vi "BuildMenu3.vi"(8 "Click Type":T6, 9 "Point":T7, 10 "XRef":refnum<vi>, 11 "State In":T10) -> (1 "Show Standard Items? (Popup click only)":bool=TRUE, 2 "Menu Specification":T9)   [LabVIEW 2012, in "CThread.lvlib" / "CThread VI Terminal Node.xnode"]
doc: "This ability VI is used to describe the menu LabVIEW will display in response to a popup (right) click or a ShowMenu reply from OperateClick.\n \n Click Type is the type of click that led to this call of the ability. Point is the location of the user's popup click, and is relative to the top-left corner of your XNode's bounds. You may use this point to make your popup sensitive to the location that was clicked. Show Standard Items? is applicable only if Click Type is Popup, and tells LabVIEW whether it should include the standard popup items that are included on every node in LabVIEW.\n \n Menu Specification is an array of clusters describing the menu.\n Item: A string that will appear in the menu.\n Id: A string that identifies this item and will be passed to SelectMenu3.\n StartSub: The current string will be the header for a pull right menu.\n EndSub: The current string will be the last item in a pull right menu.\n Checked: The current item will have a check mark next to it.\n Disabled: The current item will be diabled and greyed out.\n Separator: The current item will be a separator. Item string is not displayed.\n Help: The text that should be displayed in context help when this menu item is hovered over. This functionality is currently not implemented.\n \n The index from this array will be an input to SelectMenu3.\n \n Remember to localize the strings in your menu.\n\nDefault behavior: Only show standard items for a popup click, show nothing for operate click.\n\nThis ability does not provide UI and OS messages are not handled.\n\nSee also: SelectMenu3"
uses:
  CThread VI Terminal Node.xnode
  State.ctl
  <vilib>/XNodeSupport/XNodeMenuSpecs3.ctl
  <vilib>/XNodeSupport/XNodeMenuSpec3.ctl
  <vilib>/XNodeSupport/XNodeString.ctl
  <vilib>/XNodeSupport/XNodeBool.ctl
  <vilib>/XNodeSupport/XNodeStandardHelpInfo.ctl
  <vilib>/XNodeSupport/XNodePath.ctl
  <vilib>/XNodeSupport/XNodePoint.ctl
  <vilib>/XNodeSupport/XNodeInt.ctl
  <vilib>/XNodeSupport/XNodeClickTypes.ctl
  <vilib>/XNodeSupport/XNodeRect32.ctl
  <vilib>/XNodeSupport/NI_XNodeSupport.lvlib
panel:
  in  "Menu Item 3":T1
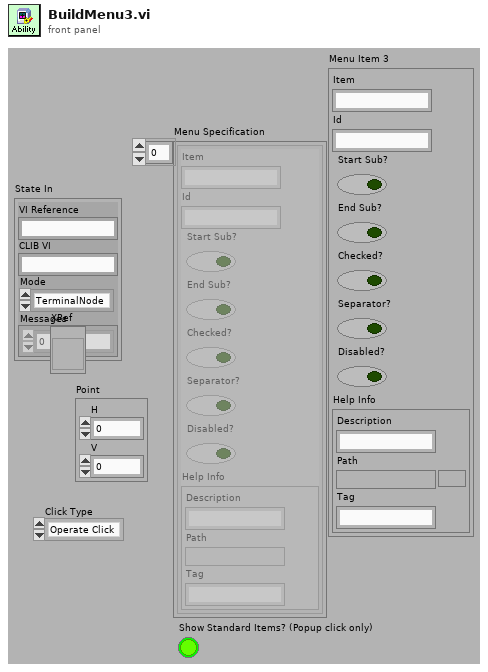
[diagram p1: front panel]
types:
  T1 = typedef "NI_XNodeSupport.lvlib/XNodeMenuSpec3.ctl" = cluster{"Item":T2, "Id":T2, "Start Sub?":T3, "End Sub?":T3, "Checked?":T3, "Separator?":T3, "Disabled?":T3, "Help Info":T4}
  T2 = typedef "NI_XNodeSupport.lvlib/XNodeString.ctl" = string
  T3 = typedef "NI_XNodeSupport.lvlib/XNodeBool.ctl" = bool
  T4 = typedef "NI_XNodeSupport.lvlib/XNodeStandardHelpInfo.ctl" = cluster{"Description":T2, "Path":T5, "Tag":T2}
  T5 = typedef "NI_XNodeSupport.lvlib/XNodePath.ctl" = path
  T6 = typedef "NI_XNodeSupport.lvlib/XNodeClickTypes.ctl" = enum32{"Operate Click", "Popup Click"}
  T7 = typedef "NI_XNodeSupport.lvlib/XNodePoint.ctl" = cluster{"H":T8, "V":T8}
  T8 = typedef "NI_XNodeSupport.lvlib/XNodeInt.ctl" = i32
  T9 = typedef "NI_XNodeSupport.lvlib/XNodeMenuSpecs3.ctl" = T1[]
  T10 = typedef "CThread.lvlib/CThread VI Terminal Node.xnode/State.ctl" = cluster{"VI Reference":string, "CLIB VI":string, "Mode":enum16{"TerminalNode", "AdaptorNode"}, "Messages":u8[]}
  T11 = typedef "NI_XNodeSupport.lvlib/XNodeRect32.ctl" = cluster{"Left":T8, "Top":T8, "Right":T8, "Bottom":T8}
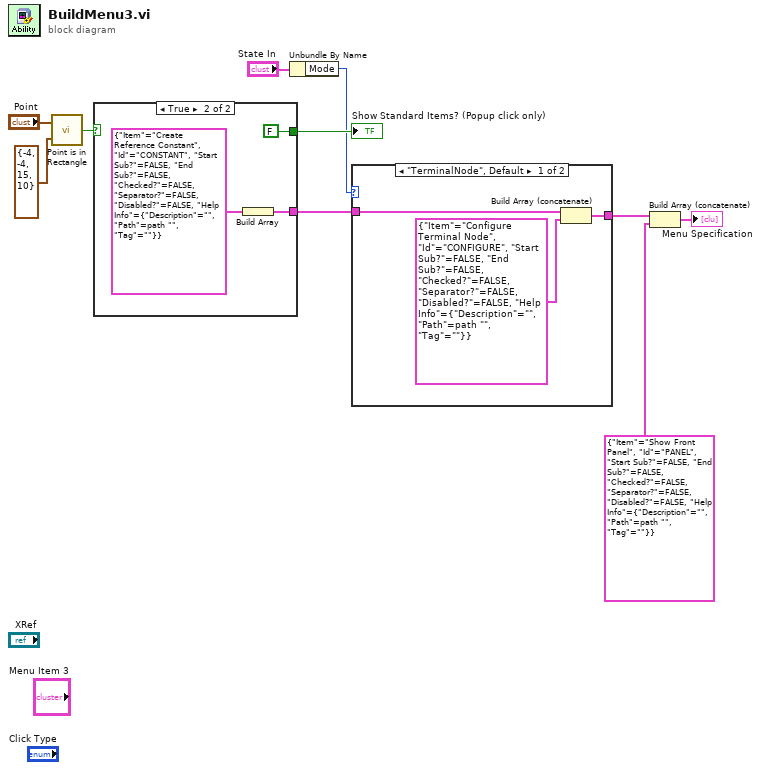
[diagram p0: block diagram]
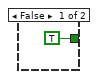
[diagram p3: hidden frame]
diagram:
  n1 = call "Point is in Rectangle.vi"("Bounds"=T11 {"Left"=-4, "Top"=-4, "Right"=15, "Bottom"=10}, "Point"="Point") -> ("In Bounds?"=w9:bool)
  n2 = case shown="True" w9 {
    tunnel: [TRUE FALSE] -> w7
    tunnel: [_ w12] -> w4
    frame False {
    }
    frame True {
      n3 = Build Array(T1 {"Item"="Create Reference Constant", "Id"="CONSTANT", "Start Sub?"=FALSE, "End Sub?"=FALSE, "Checked?"=FALSE, "Separator?"=FALSE, "Disabled?"=FALSE, "Help Info"={"Description"="", "Path"=path "", "Tag"=""}} ("Menu Item 3")) -> (w12:T1[])
    }
  }
  "Show Standard Items? (Popup click only)" <- w7
  n4 = Unbundle By Name("State In") -> ("Mode"=w5:enum16{"TerminalNode", "AdaptorNode"})
  n5 = case shown="\"TerminalNode\", Default" w5 {
    tunnel: w4 -> [w17 w18]
    tunnel: [w15 w18] -> w3
    frame "TerminalNode", Default {
      n6 = Build Array (concatenate)(w17, T1 {"Item"="Configure Terminal Node", "Id"="CONFIGURE", "Start Sub?"=FALSE, "End Sub?"=FALSE, "Checked?"=FALSE, "Separator?"=FALSE, "Disabled?"=FALSE, "Help Info"={"Description"="", "Path"=path "", "Tag"=""}} ("Menu Item 3")) -> (w15:T1[])
    }
    frame "AdaptorNode" {
    }
  }
  n7 = Build Array (concatenate)(w3, T1 {"Item"="Show Front Panel", "Id"="PANEL", "Start Sub?"=FALSE, "End Sub?"=FALSE, "Checked?"=FALSE, "Separator?"=FALSE, "Disabled?"=FALSE, "Help Info"={"Description"="", "Path"=path "", "Tag"=""}} ("Menu Item 3")) -> (→"Menu Specification":T1[])
